vi "Read VI Ref.vi"(8 "error in (no error)":errorcluster, 11 "CSM-Helper in":refnum<class "CSM-Helper.lvclass">) -> (0 "error out":errorcluster, 2 "VI":refnum<vi>, 3 "CSM-Helper out":refnum<class "CSM-Helper.lvclass">)   [LabVIEW 2020, in "CSM-Helper.lvclass"]
uses:
  CSM-Helper.lvclass
  CSM-Helper.lvclass/CSM-Helper.ctl
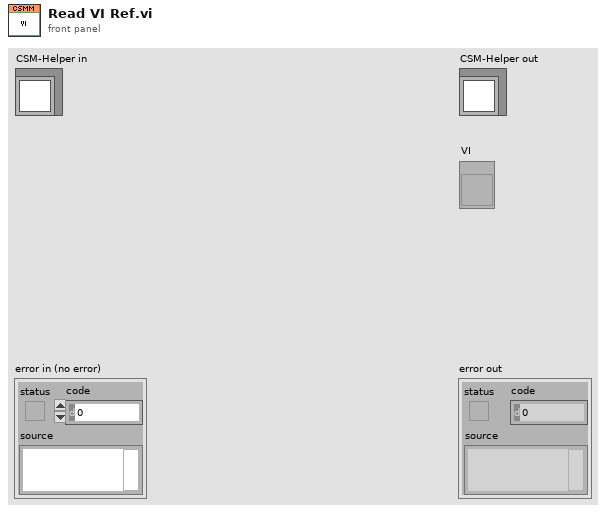
[diagram p1: front panel]
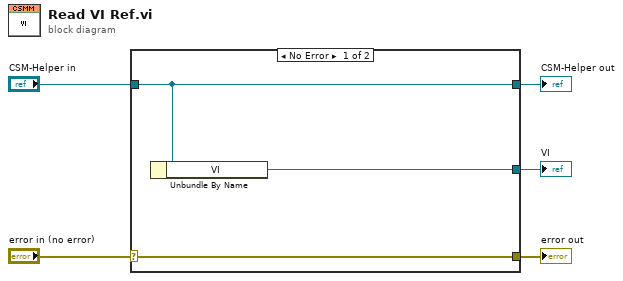
[diagram p0: block diagram]
diagram:
  n1 = case shown="No Error" "error in (no error)" {
    selector: "error in (no error)" -> [w8 w9]
    tunnel: [w8 w9] -> w4
    tunnel: [w7 w10] -> w2
    tunnel: "CSM-Helper in" -> [w7 w10]
    tunnel: [w6 _] -> w1
    frame No Error {
      n2 = Unbundle By Name(w7) -> ("VI"=w6:refnum<vi>)
    }
    frame Error {
    }
  }
  "error out" <- w4
  "CSM-Helper out" <- w2
  "VI" <- w1
